vi "test Execute.vi"(8 "error in (no error)":errorcluster, 11 "TestCase in":refnum<class "Single Consumer Test Case.lvclass">) -> (0 "error out":errorcluster, 3 "TestCase out":refnum<class "Single Consumer Test Case.lvclass">)   [LabVIEW 2027, in "Single Consumer Test Case.lvclass"]
uses:
  Single Consumer Test Case.lvclass
  Support/Messages/Test Message/Test Message.lvclass
  C:/NetCore/niveristand-custom-device-message-library/Source/Message/Abstract Message/Abstract Message.lvclass
  Message/Shutdown Message/Shutdown Message.lvclass
  Support/Message String Action.ctl
  Single Consumer Test Case.lvclass/Single Consumer Test Case.ctl
  Producer/Abstract Producer/Abstract Producer.lvclass
  C:/Program Files/National Instruments/LabVIEW 2027/vi.lib/addons/_JKI Toolkits/VI Tester/TestCase.llb/TestCase.lvclass
  <vilib>/addons/_JKI Toolkits/VI Tester/TestCase.llb/TestCase.lvclass
  Consumer/Abstract Consumer/Abstract Consumer.lvclass
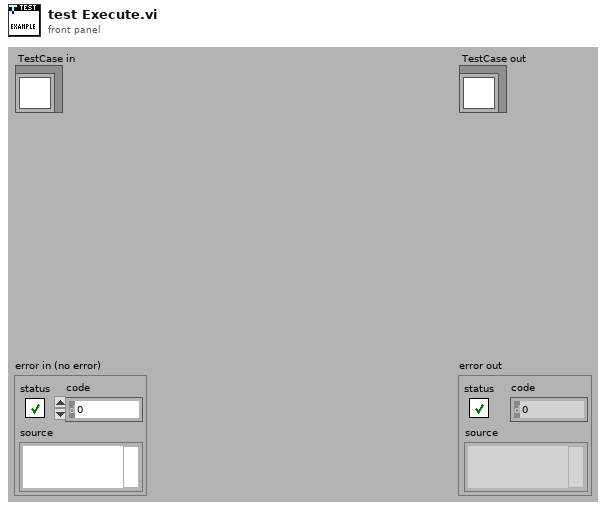
[diagram p1: front panel]
types:
  T1 = typedef "Message String Action.ctl" = enum16{"Get String", "Set String", "Reset"}
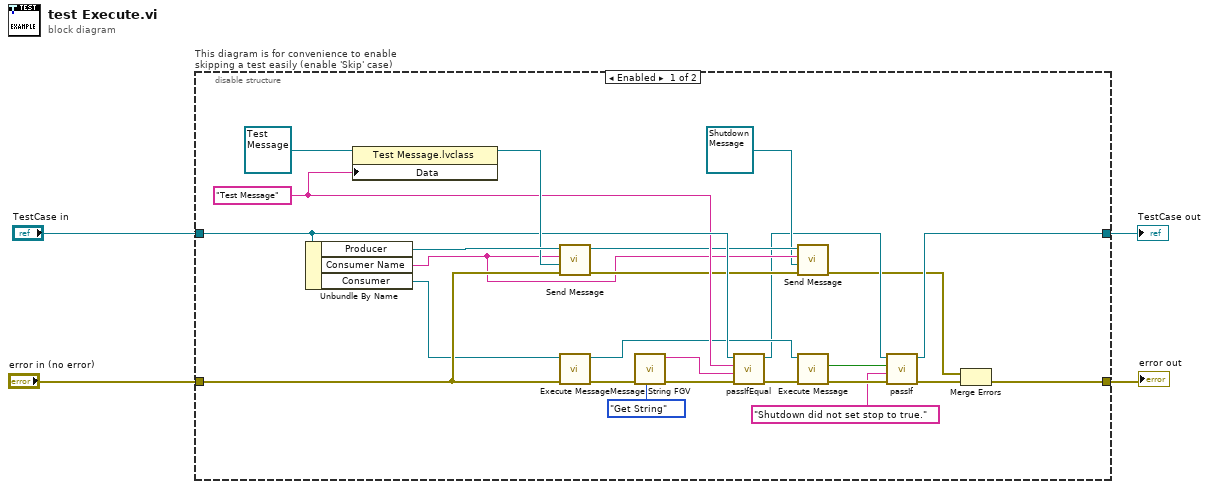
[diagram p0: block diagram]
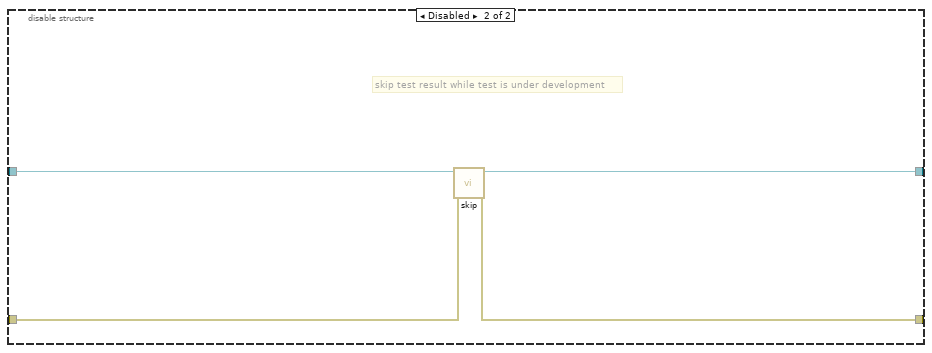
[diagram p2: hidden frame]
diagram:
  n1 = disable-structure "This diagram is for convenience to enable skipping a test easily (enable 'Skip' case)" shown="Enabled" {
    disable-tunnel: "TestCase in" -> [w23 w33]
    disable-tunnel: [w10 w31] -> w1
    disable-tunnel: [w6 w32] -> w3
    disable-tunnel: "error in (no error)" -> [w29 w30]
    frame Enabled {
      w21 = "Test Message" ("Data")
      n2 = Unbundle By Name(w23) -> ("Producer"=w27:refnum<class "Abstract Producer.lvclass">, "Consumer Name"=w18:string, "Consumer"=w28:refnum<class "Abstract Consumer.lvclass">)
      n3 = property class="Test Message.lvclass"(reference=refnum<class "Test Message.lvclass"> refnum ("Test Message.lvclass"), "Data"=w21) -> (reference out=w26:refnum<class "Test Message.lvclass">)  [unwired: 1 in, 1 out]
      n4 = call-dynamic "Send Message.vi"("error in (no error)"=w29, "Message in"=w26, "Consumer in"=w18, "Abstract Producer in"=w27) -> ("error out"=w20:errorcluster, "Abstract Producer out"=w19:refnum<class "Abstract Producer.lvclass">)  [unwired: 4 in, 2 out]
      n5 = call "Execute Message.vi"("error in (no error)"=w29, "Abstract Consumer in"=w28) -> ("error out"=w25:errorcluster, "Abstract Consumer out"=w15:refnum<class "Abstract Consumer.lvclass">)  [unwired: 6 in, 2 out]
      n6 = call "Message String FGV.vi"("Action"=Message_String_Action."Get String", "error in (no error)"=w25) -> ("error out"=w24:errorcluster, "String out"=w22:string)  [unwired: 8 in]
      n7 = call-dynamic "passIfEqual.vi"("error in (no error)"=w24, "y"=w22, "x"=w21, "TestCase in"=w23) -> ("error out"=w16:errorcluster, "TestCase out"=w11:refnum<class "Single Consumer Test Case.lvclass">)  [unwired: 6 in]
      n8 = call-dynamic "Send Message.vi"("error in (no error)"=w20, "Message in"=refnum<class "Shutdown Message.lvclass"> refnum ("Messaging.lvlib:Message.lvlib:Shutdown Message.lvclass"), "Consumer in"=w18, "Abstract Producer in"=w19) -> ("error out"=w8:errorcluster)  [unwired: 4 in, 3 out]
      n9 = call "Execute Message.vi"("error in (no error)"=w16, "Abstract Consumer in"=w15) -> ("error out"=w14:errorcluster, "Stop?"=w13:bool)  [unwired: 6 in, 2 out]
      n10 = call-dynamic "passIf.vi"("error in (no error)"=w14, "message (\"\")"="Shutdown did not set stop to true." ("message (\"\")"), "pass"=w13, "TestCase in"=w11) -> ("error out"=w9:errorcluster, "TestCase out"=w10:refnum<class "Single Consumer Test Case.lvclass">)  [unwired: 6 in]
      n11 = Merge Errors(w8, w9) -> (w6:errorcluster)
    }
    frame Disabled {
      # "skip test result while test is under development"
      n12 = call <vilib>:"skip.vi"("error in (no error)"=w30, "TestCase in"=w33) -> ("error out"=w32:errorcluster, "TestCase out"=w31:refnum<class "Single Consumer Test Case.lvclass">)  [unwired: 8 in]
    }
  }
  "error out" <- w3
  "TestCase out" <- w1
